vi "IMAQDevice.setTriggerMode.vi"(0 "i ref in":refnum<vi>, 2 "TriggerMode":i32, 5 "error in (no error)":errorcluster) -> (14 "i ref out":refnum<vi>, 19 "error out":errorcluster)   [LabVIEW 2014, in "IMAQDevice.lvlib"]
doc: "This VI allows to change the trigger mode of the camera. The explicit meaning of the different values depends on the used camera and can therefore vary.\n\nLicense Agreement for this software:\n\nCopyright (C)\nGesellschaft für Schwerionenforschung, GSI\nPlanckstr. 1\n64291 Darmstadt\nGermany\n\nContact: D.Beck@gsi.de \n\nThis program is free software; you can redistribute it and/or modify it under the terms of the \nGNU General Public License as published by the Free Software Foundation; either version 2 of \nthe license, or (at your option) any later version.\n\nThis program is distributed in the hope that it will be useful, but WITHOUT ANY WARRANTY; \nwithout even the implied warranty of MERCHANTABILITY or FITNESS FOR A PARTICULAR PURPOSE. See the GNU General License for more details (http://www.gnu.org).\n\nGesellschaft für Schwerionenforschung, GSI\nPlanckstr. 1, 64291 Darmstadt, Germany\nFor all questions and ideas contact: M.Richter@gsi.de, H.Brand@gsi.de or D.Beck@gsi.de.\nLast update: 16-JUN-2004"
uses:
  IMAQDevice.lvlib
  CSlibraries-extern/DimLVEvent/LVDimInterface/LVDimInterface.lvlib
  CSlibraries-extern/HGF/HGF_LVC/HGF_IMAQ/HGF_IMAQDevice/HGF_IMAQDevice.lvclass
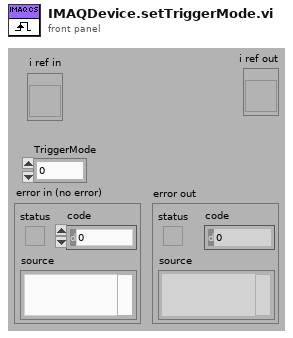
[diagram p1: front panel]
types:
  T1 = typedef "IMAQDevice.lvlib/IMAQDevice.i attribute.ctl" = cluster{"HGF_IMAQ.lvlib:HGF_IMAQDevice.lvclass":refnum<class "HGF_IMAQDevice.lvclass">, "Image":T2, "TimeStampID":i32, "Image IDs":i32[], "NumberOfImagesID":i32, "JPEG?":bool, "JPEGID":i32, "JPEG_ImageID":i32, "TriggerModeID":i32, "OffsetFromLeft":i32, "OffsetFromTop":i32, "HorizontalPixelPerMm":dbl, "VerticalPixelPerMm":dbl, "Grid":cluster{"1":cluster{i32, i32}, "2":cluster{i32, i32}, "3":cluster{i32, i32}, "4":cluster{i32, i32}}, "GridR":cluster{"1":cluster{dbl, dbl}, "2":cluster{dbl, dbl}, "3":cluster{dbl, dbl}, "4":cluster{dbl, dbl}}, "CameraTypeID":i32, "CameraInfos":cluster{"Camera Name-Array":string[], "own Camera Type":string}, "TakeMeasurement?":bool, "TriggerArmedID":i32, "Mirroring":i16, "Rotation":dbl}
  T2 = typedef "IMAQ Image.ctl" = refnum<image>
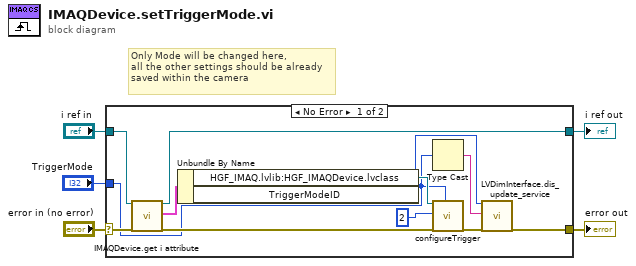
[diagram p0: block diagram]
diagram:
  # "Only Mode will be changed here,\nall the other settings should be already\nsaved within the camera"
  n1 = case shown="No Error" "error in (no error)" {
    selector: "error in (no error)" -> [w16 w19]
    tunnel: "i ref in" -> [w17 w18]
    tunnel: [w15 w19] -> w3
    tunnel: [w11 w18] -> w2
    tunnel: "TriggerMode" -> [w7 _]
    frame No Error {
      n2 = call "IMAQDevice.get i attribute.vi"("i ref in"=w17, "error in (no error)"=w16) -> ("i ref out"=w11:refnum<vi>, "i attribute"=w14:T1, "error out"=w9:errorcluster)  [unwired: 15 in]
      n3 = Unbundle By Name(w14) -> ("HGF_IMAQ.lvlib:HGF_IMAQDevice.lvclass"=w8:refnum<class "HGF_IMAQDevice.lvclass">, "TriggerModeID"=w13:i32)
      n4 = Type Cast(x=w7) -> (*(type *) &x=w12:string)  [unwired: 1 in]
      n5 = call "configureTrigger.vi"("HGF_IMAQDevice"=w8, "Line Number (0)"=u32 2, "error in (no error)"=w9, "Mode (off)"=w7) -> ("error out"=w10:errorcluster)  [unwired: 14 in, 1 out]
      n6 = call "LVDimInterface.dis_update_service.vi"("my_serviceID"=w13, "data"=w12, "error in (no error)"=w10) -> ("error out"=w15:errorcluster)  [unwired: 14 in, 2 out]
    }
    frame Error {
    }
  }
  "i ref out" <- w2
  "error out" <- w3
